vi "Flash parameters.vi"() -> ()   [LabVIEW 2016]
uses:
  Set Load Default Object Dictionary.vi
  Set Save Object Dictionary.vi
  <vilib>/CANopenLib/CANOPEN.llb/CANopen SDO Create.vi
  <vilib>/CANopenLib/CANOPEN.llb/CANopen SDO Write.vi
  <vilib>/CANopenLib/CANOPEN.llb/CANopen SDO Write [STR].vi
  <vilib>/CANopenLib/CANOPEN.llb/CANopen SDO Close.vi
  <vilib>/CANopenLib/CANOPEN.llb/CANopen Interface Close.vi
panel:
  out "Reset controler":bool
  in  "?":bool
  out "description":string
  out "completion code 3":u32
  out "completion code 2":u32
  out "completion code":u32
  in  "Motor":u8(ring) items=["Right", "Left"]
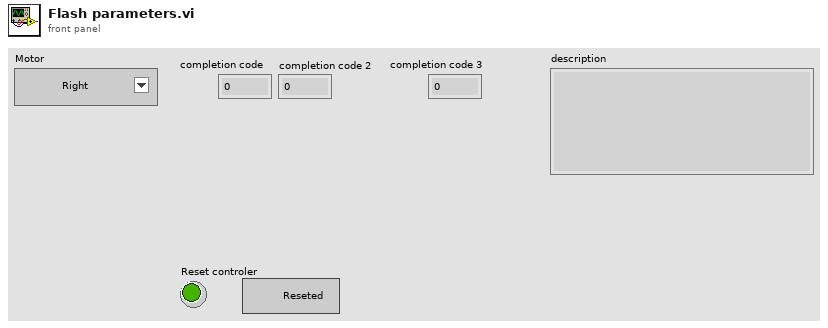
[diagram p1: front panel]
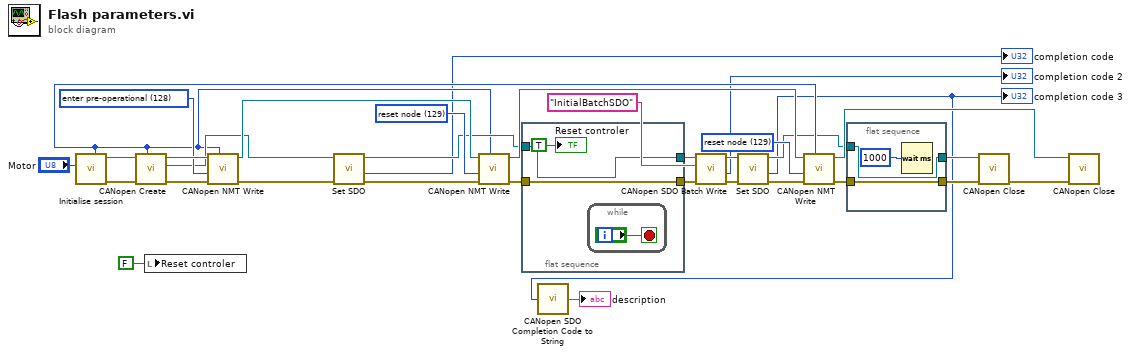
[diagram p0: block diagram]
diagram:
  w12 = u16 129 items=["start remote node"=1, "stop remote node"=2, "enter pre-operational"=128, "reset node"=129, "reset communication"=130] ("command")
  w21 = u16 129 items=["start remote node"=1, "stop remote node"=2, "enter pre-operational"=128, "reset node"=129, "reset communication"=130] ("command")
  w24 = u16 128 items=["start remote node"=1, "stop remote node"=2, "enter pre-operational"=128, "reset node"=129, "reset communication"=130] ("command")
  n1 = call "Initialise session.vi"("Motor"="Motor") -> ("error out"=w32:errorcluster, "interface object out"=w31:refnum<k20>, "Used Node ID"=w10:u8)  [unwired: 8 in]
  n2 = call-poly <vilib>:"CANopen Create.vi"("node-ID"=w10, "error in (no error)"=w32, "interface object in"=w31) -> ("error out"=w26:errorcluster, "SDO object out"=w11:refnum<k20>, "interface object out"=w27:refnum<k20>)  [unwired: 6 in]
  n3 = local write "Reset controler"(FALSE ("Reset controler")) -> ()
  n4 = call <vilib>:"CANopen NMT Write.vi"("node-ID (0)"=w10, "error in (no error)"=w26, "command"=w24, "interface object in"=w27) -> ("error out"=w25:errorcluster, "interface object out"=w20:refnum<k20>)  [unwired: 6 in]
  n5 = call-poly "Set SDO.vi"("error in (no error)"=w25, "SDO object in"=w11) -> ("error out"=w22:errorcluster, "completion code"=→"completion code":u32, "SDO object out"=w14:refnum<k20>)  [unwired: 7 in]
  n6 = call <vilib>:"CANopen NMT Write.vi"("node-ID (0)"=w10, "error in (no error)"=w22, "command"=w21, "interface object in"=w20) -> ("error out"=w23:errorcluster, "interface object out"=w19:refnum<k20>)  [unwired: 6 in]
  n7 = flat-sequence {
    tunnel: [w36] -> w28
    tunnel: w23 -> [w36]
    tunnel: w14 -> [w35]
    tunnel: [w35] -> w13
    frame #0 {
      n8 = while {
        stop <- "?" stop-if-true
      }
      "Reset controler" <- TRUE ("Reset controler")
    }
  }
  n9 = call <vilib>:"CANopen SDO Batch Write.vi"("error in (no error)"=w28, "batch SDO name"="InitialBatchSDO", "SDO object in"=w13) -> ("error out"=w5:errorcluster, "completion code"=→"completion code 2":u32, "SDO object out"=w9:refnum<k20>)  [unwired: 6 in]
  n10 = call-poly "Set SDO.vi"("error in (no error)"=w5, "SDO object in"=w9) -> ("error out"=w7:errorcluster, "completion code"=w1:u32, "SDO object out"=w8:refnum<k20>)  [unwired: 7 in]
  "completion code 3" <- w1
  n11 = call <vilib>:"CANopen SDO Completion Code to String.vi"("SDO completion code"=w1) -> ("description"=→"description":string)
  n12 = call <vilib>:"CANopen NMT Write.vi"("node-ID (0)"=w10, "error in (no error)"=w7, "command"=w12, "interface object in"=w19) -> ("error out"=w15:errorcluster, "interface object out"=w18:refnum<k20>)  [unwired: 6 in]
  n13 = flat-sequence {
    tunnel: [w39] -> w17
    tunnel: w8 -> [w39]
    tunnel: [w38] -> w16
    tunnel: w15 -> [w38]
    frame #0 {
      n14 = Wait (ms)(milliseconds to wait=u32 1000) -> ()  [unwired: 1 out]
    }
  }
  n15 = call-poly <vilib>:"CANopen Close.vi"("error in (no error)"=w16, "SDO object in"=w17) -> ("error out"=w30:errorcluster)  [unwired: 9 in]
  n16 = call-poly <vilib>:"CANopen Close.vi"("error in (no error)"=w30, "interface object in"=w18) -> ()  [unwired: 9 in, 1 out]
